vi "Init from Timestamp.vi"(8 "error in":errorcluster, 10 "Timestamp":timestamp format="%<%x %.3X>T", 11 "Timestamp in":refnum<class "Timestamp.lvclass">) -> (0 "error out":errorcluster, 3 "Timestamp out":refnum<class "Timestamp.lvclass">)   [LabVIEW 2024, in "Timestamp.lvclass"]
uses:
  Timestamp.lvclass
  Timestamp.lvclass/Timestamp.ctl
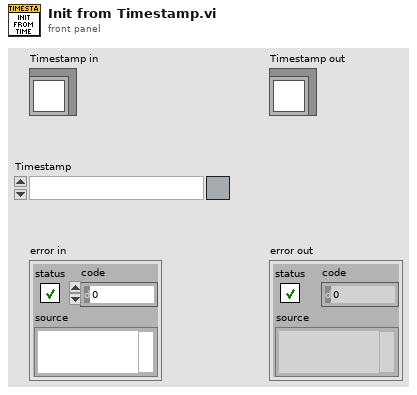
[diagram p1: front panel]
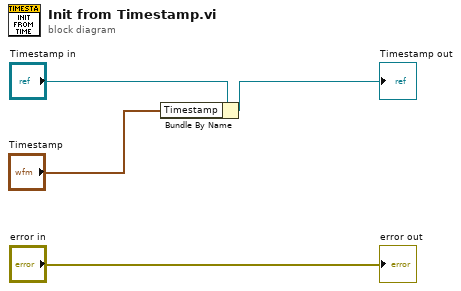
[diagram p0: block diagram]
diagram:
  n1 = Bundle By Name(cluster="Timestamp in", "Timestamp"="Timestamp") -> (→"Timestamp out":refnum<class "Timestamp.lvclass">)
  "error out" <- "error in"
